vi "Measurement-RT.vi"(1 "Ctl Refnum 2":refnum<vi>, 2 "Ctl Refnum":refnum<vi>, 8 "error in (no error)":errorcluster, 9 "BSFR":refnum<file>, 10 "Cluster 2":T3, 11 "簇":cluster{"开始温度":dbl, "结束温度":dbl, "变温速率":dbl}) -> (7 "Cluster":T1)   [LabVIEW 2017]
uses:
  <vilib>/Instr/_visa.llb/VISA Configure Serial Port (Instr).vi
panel:
  out "电抗":dbl
  out "电阻":dbl
  in  "Cluster 3":T2
  in  "高温&低温":u16(ring) items=["低温", "高温"]
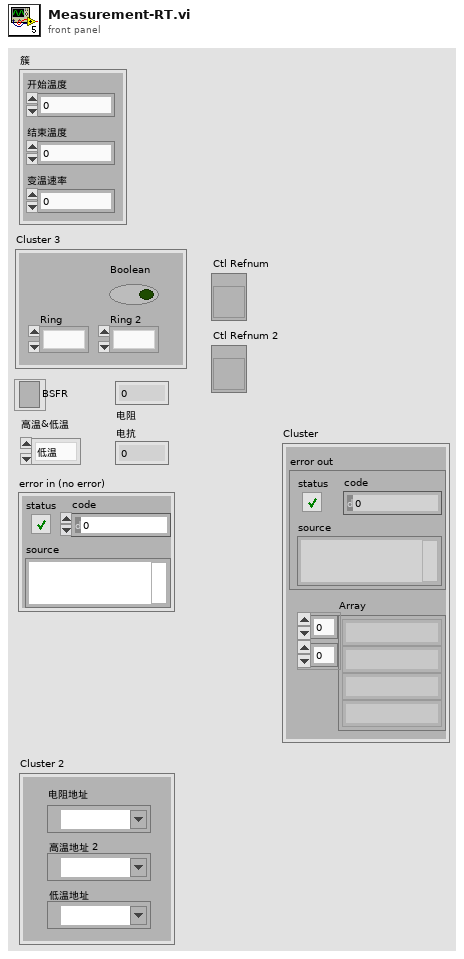
[diagram p1: front panel]
types:
  T1 = cluster{"Array":string[][], "error out":errorcluster}
  T2 = cluster{"Boolean":bool, "Ring":u16, "Ring 2":u16}
  T3 = cluster{"电阻地址":refnum<visa-resource-name>, "低温地址":refnum<visa-resource-name>, "高温地址 2":refnum<visa-resource-name>}
  T4 = cluster{"Array 2":string[][], "error out":errorcluster}
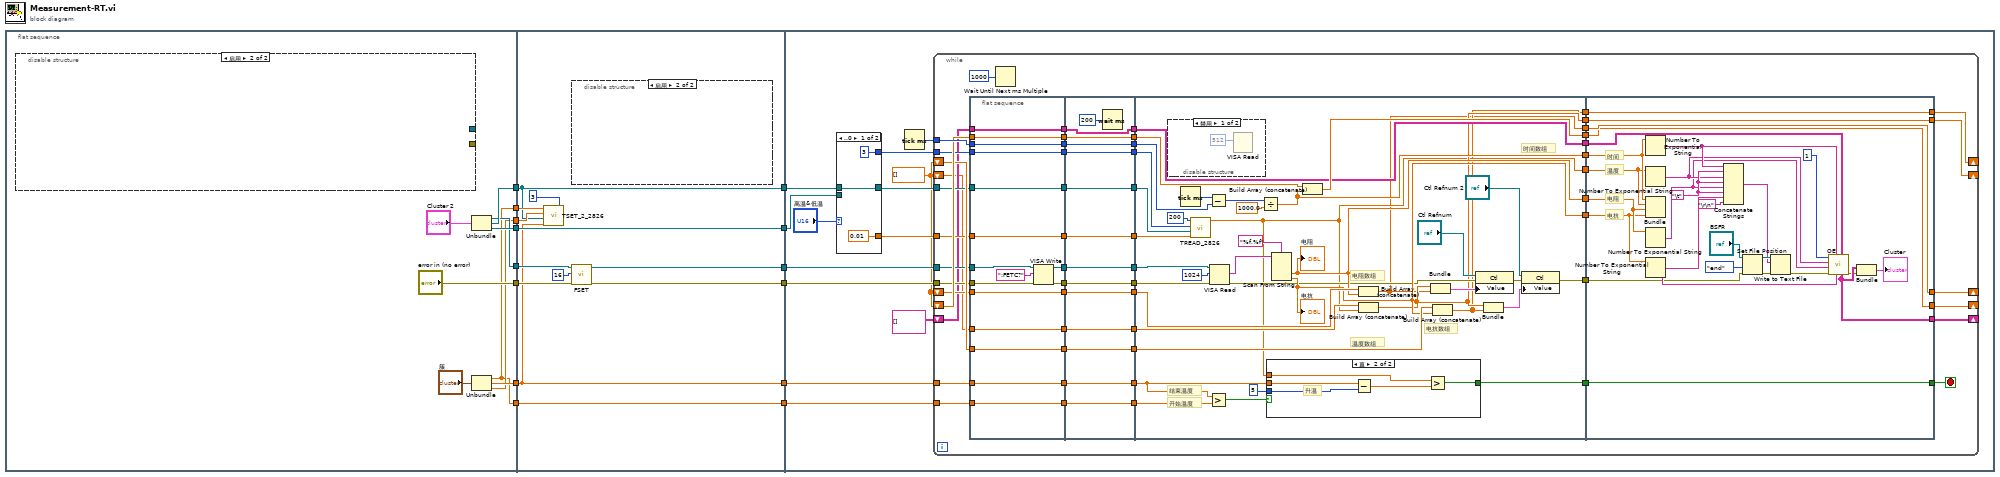
[diagram p0: block diagram]
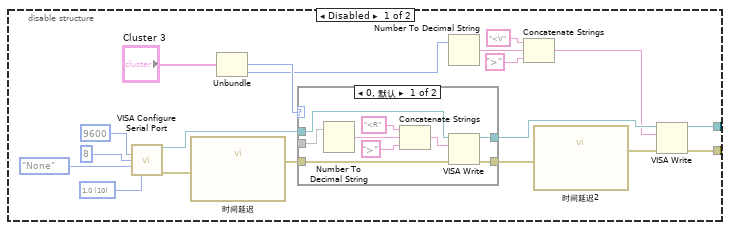
[diagram p2: hidden frame]
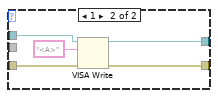
[diagram p3: hidden frame]
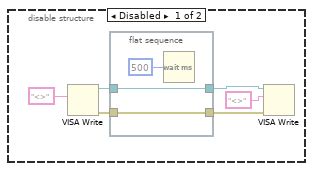
[diagram p4: hidden frame]
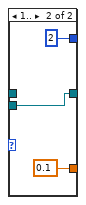
[diagram p5: hidden frame]
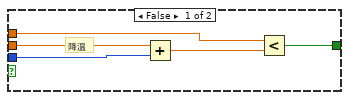
[diagram p6: hidden frame]
diagram:
  n1 = flat-sequence {
    tunnel: [w22] -> w10
    tunnel: [w21] -> w9
    tunnel: [w19] -> w7
    tunnel: ["error in (no error)"] -> w6
    tunnel: [w17] -> w5
    tunnel: [w15] -> w4
    tunnel: [w16] -> w3
    tunnel: [w15] -> w1
    tunnel: [w59] -> w14
    tunnel: [w66] -> w13
    tunnel: [w58] -> w12
    tunnel: [w62] -> w11
    tunnel: w10 -> [w58]
    tunnel: w9 -> [w62]
    tunnel: [w64] -> w8
    tunnel: w7 -> [w67]
    tunnel: w6 -> [w65]
    tunnel: w5 -> [w59]
    tunnel: w4 -> [w61]
    tunnel: w3 -> [w60]
    tunnel: [w57] -> w2
    tunnel: w1 -> [w57]
    tunnel: w14 -> [w85]
    tunnel: w13 -> [w84]
    tunnel: w12 -> [w83]
    tunnel: w11 -> [w82]
    tunnel: w8 -> [w81]
    tunnel: w2 -> [w78]
    frame #0 {
      n2 = disable-structure shown="启用" {
        disable-tunnel: [w27 _] -> _
        disable-tunnel: [w26 _] -> _
        frame Disabled {
          w39 = u16 10 items=["1.0"=10, "1.5"=15, "2.0"=20] ("stop bits (10: 1 bit)")
          n3 = call-poly "VISA Configure Serial Port"("baud rate (9600)"=u32 9600, "data bits (8)"=u16 8, "parity (0:none)"=enum16{"None", "Odd", "Even", "Mark", "Space"}."None", "stop bits (10: 1 bit)"=w39) -> ("VISA resource name out"=w37:refnum<visa-resource-name>, "error out"=w31:errorcluster)  [unwired: 10 in]
          n4 = call "时间延迟"("error in (no error)"=w31) -> ("error out"=w30:errorcluster)  [unwired: 10 in]
          n5 = Unbundle("Cluster 3") -> ("Ring"=w25:u16, "Ring 2"=w24:u16)  [unwired: 1 out]
          n6 = case shown="0, 默认" w25 {
            tunnel: w37 -> [w51 w56]
            tunnel: _ -> [w48 _]
            tunnel: w30 -> [w45 w54]
            tunnel: [w44 w53] -> w36
            tunnel: [w43 w52] -> w28
            frame 0, Default {
              n7 = Number To Decimal String(number=w48) -> (decimal integer string=w47:string)  [unwired: 1 in]
              n8 = Concatenate Strings("<R" ("字符串"), w47, ">" ("字符串")) -> (w46:string)
              n9 = VISA Write(VISA resource name=w51, write buffer=w46, error in (no error)=w45) -> (VISA resource name out=w44:refnum<visa-resource-name>, error out=w43:errorcluster)  [unwired: 1 out]
            }
            frame 1 {
              n10 = VISA Write(VISA resource name=w56, write buffer="<A>" ("写入缓冲区"), error in (no error)=w54) -> (VISA resource name out=w53:refnum<visa-resource-name>, error out=w52:errorcluster)  [unwired: 1 out]
            }
          }
          n11 = Number To Decimal String(number=w24) -> (decimal integer string=w33:string)  [unwired: 1 in]
          n12 = Concatenate Strings("<V" ("字符串"), w33, ">" ("字符串")) -> (w32:string)
          n13 = call "时间延迟2"("error in (no error)"=w28) -> ("error out"=w29:errorcluster)  [unwired: 10 in]
          n14 = VISA Write(VISA resource name=w36, write buffer=w32, error in (no error)=w29) -> (VISA resource name out=w27:refnum<visa-resource-name>, error out=w26:errorcluster)  [unwired: 1 out]
        }
        frame Enabled {
        }
      }
      n15 = Unbundle("Cluster 2") -> ("电阻地址"=w19:refnum<visa-resource-name>, "低温地址"=w22:refnum<visa-resource-name>, "高温地址 2"=w21:refnum<visa-resource-name>)
      n16 = Unbundle("簇") -> ("开始温度"=w15:dbl, "结束温度"=w17:dbl, "变温速率"=w16:dbl)
    }
    frame #1 {
      n17 = call "TSET_2_2826.vi"("Address No."=i8 3, "T-Ending, C"=w59, "VISA resource name"=w58, "cooling/heating rate, C/min"=w60, "T-Starting, C"=w61) -> ()
      n18 = disable-structure shown="启用" {
        frame Disabled {
          n19 = VISA Write(write buffer="<>" ("写入缓冲区")) -> (VISA resource name out=w73:refnum<visa-resource-name>, error out=w71:errorcluster)  [unwired: 2 in, 1 out]
          n20 = flat-sequence {
            tunnel: w73 -> [w76]
            tunnel: [w76] -> w72
            tunnel: w71 -> [w75]
            tunnel: [w75] -> w70
            frame #0 {
              n21 = Wait (ms)(milliseconds to wait=u32 500 ("等待时间（毫秒）")) -> ()  [unwired: 1 out]
            }
          }
          n22 = VISA Write(VISA resource name=w72, write buffer="<>" ("写入缓冲区"), error in (no error)=w70) -> ()  [unwired: 3 out]
        }
        frame Enabled {
        }
      }
      n23 = call "FSET.vi"("error in (no error)"=w65, "Function (0: Cp-D)"=16, "VISA resource name"=w67) -> ("error out"=w64:errorcluster, "VISA resource name out"=w66:refnum<visa-resource-name>)  [unwired: 7 in]
    }
    frame #2 {
      w79 = dbl[] []
      n24 = case shown="..0" "高温&低温" {
        tunnel: [w91 w94] -> w88
        tunnel: [3 2] -> w87
        tunnel: [0.01 0.1] -> w86
        tunnel: w83 -> [w91 _]
        tunnel: w82 -> [_ w94]
        frame ..0 {
        }
        frame 1.. {
        }
      }
      n25 = Tick Count (ms)() -> (millisecond timer value=w90:u32)
      n26 = while {
        tunnel: w90 -> [w153]
        shift-right: [w146] -> _
        shift-left: w79 -> [w151]
        shift-right: [w147] -> _
        shift-left: w79 -> [w150]
        shift-right: [w148] -> _
        shift-left: w79 -> [w149]
        tunnel: w88 -> [w137]
        tunnel: w87 -> [w136]
        tunnel: w86 -> [w135]
        tunnel: w85 -> [w133]
        tunnel: w84 -> [w132]
        tunnel: w81 -> [w131]
        shift-right: [w109] -> _
        shift-left: string[][] [] -> [w105]
        shift-right: [w104] -> _
        shift-left: w79 -> [w100]
        tunnel: w78 -> [w99]
        stop <- w152 stop-if-true
        n27 = flat-sequence {
          tunnel: w131 -> [w157]
          tunnel: w133 -> [w162]
          tunnel: w132 -> [w160]
          tunnel: w135 -> [w163]
          tunnel: w136 -> [w164]
          tunnel: w137 -> [w165]
          tunnel: w149 -> [w166]
          tunnel: w150 -> [w167]
          tunnel: w151 -> [w168]
          tunnel: w153 -> [w169]
          tunnel: [w169] -> w130
          tunnel: [w168] -> w128
          tunnel: [w167] -> w126
          tunnel: [w166] -> w124
          tunnel: [w165] -> w122
          tunnel: [w164] -> w120
          tunnel: [w163] -> w118
          tunnel: [w159] -> w116
          tunnel: [w162] -> w114
          tunnel: [w158] -> w112
          tunnel: [w156] -> w106
          tunnel: w105 -> [w156]
          tunnel: [w155] -> w101
          tunnel: w100 -> [w155]
          tunnel: w99 -> [w154]
          tunnel: [w154] -> w97
          tunnel: w130 -> [w183]
          tunnel: [w183] -> w129
          tunnel: w128 -> [w182]
          tunnel: [w182] -> w127
          tunnel: w126 -> [w181]
          tunnel: [w181] -> w125
          tunnel: w124 -> [w180]
          tunnel: [w180] -> w123
          tunnel: w122 -> [w179]
          tunnel: [w179] -> w121
          tunnel: w120 -> [w178]
          tunnel: [w178] -> w119
          tunnel: w118 -> [w177]
          tunnel: [w177] -> w117
          tunnel: w116 -> [w176]
          tunnel: [w176] -> w115
          tunnel: w114 -> [w175]
          tunnel: [w175] -> w113
          tunnel: w112 -> [w174]
          tunnel: [w174] -> w111
          tunnel: [w172] -> w107
          tunnel: w106 -> [w172]
          tunnel: [w171] -> w102
          tunnel: w101 -> [w171]
          tunnel: [w170] -> w98
          tunnel: w97 -> [w170]
          tunnel: [w190] -> w145
          tunnel: [w185] -> w144
          tunnel: [w186] -> w143
          tunnel: [w214] -> w142
          tunnel: [w207] -> w141
          tunnel: [w206] -> w140
          tunnel: [w213] -> w139
          tunnel: [w184] -> w138
          tunnel: [w188] -> w134
          tunnel: w129 -> [w220]
          tunnel: w127 -> [w217]
          tunnel: w125 -> [w216]
          tunnel: w123 -> [w215]
          tunnel: w121 -> [w212]
          tunnel: w119 -> [w210]
          tunnel: w117 -> [w209]
          tunnel: w115 -> [w197]
          tunnel: w113 -> [w189]
          tunnel: w111 -> [w196]
          tunnel: [w195] -> w108
          tunnel: w107 -> [w195]
          tunnel: [w194] -> w103
          tunnel: w102 -> [w193]
          tunnel: w98 -> [w192]
          tunnel: [w255] -> w152
          tunnel: w145 -> [w255]
          tunnel: [w254] -> w148
          tunnel: w144 -> [w254]
          tunnel: [w253] -> w147
          tunnel: w143 -> [w253]
          tunnel: [w252] -> w146
          tunnel: w142 -> [w252]
          tunnel: w141 -> [w246]
          tunnel: w140 -> [w245]
          tunnel: w139 -> [w248]
          tunnel: w138 -> [w236]
          tunnel: w134 -> [w247]
          tunnel: [w237] -> w109
          tunnel: w108 -> [w239]
          tunnel: [w233] -> w104
          tunnel: w103 -> [w233]
          frame #0 {
            n28 = VISA Write(VISA resource name=w160, write buffer=":FETC?", error in (no error)=w157) -> (VISA resource name out=w159:refnum<visa-resource-name>, error out=w158:errorcluster)  [unwired: 1 out]
          }
          frame #1 {
            n29 = Wait (ms)(milliseconds to wait=u32 200 ("等待时间（毫秒）")) -> ()  [unwired: 1 out]
          }
          frame #2 {
            # "开始温度"
            # "结束温度"
            # "温度数组"
            # "电阻数组"
            # "电抗数组"
            # "时间数组"
            n30 = disable-structure shown="禁用" {
              frame Disabled {
                n31 = VISA Read(byte count=u32 512 ("字节总数")) -> ()  [unwired: 2 in, 4 out]
              }
              frame Enabled {
              }
            }
            n32 = Tick Count (ms)() -> (millisecond timer value=w221:u32)
            n33 = call "TREAD_2826.vi"("Unknown Param 2"=w209, "VISA resource name"=w212, "Address No."=w210, "Unknown Param"=200) -> ("PV"=w188:dbl)  [unwired: 3 out]
            n34 = Subtract(x=w221, y=w220) -> (x-y=w219:u32)
            n35 = Greater?(x=w189, y=w192) -> (0:w191:bool)
            n36 = VISA Read(VISA resource name=w197, byte count=1024, error in (no error)=w196) -> (read buffer=w199:string, error out=w198:errorcluster)  [unwired: 2 out]
            n37 = Divide(x=w219, y=1000.0) -> (x/y=w213:dbl)
            n38 = case shown="真" w191 {
              tunnel: [w223 w230] -> w190
              tunnel: w189 -> [w226 w229]
              tunnel: w188 -> [w225 w231]
              tunnel: 5 -> [w222 w228]
              frame False {
                # "降温"
                n39 = Add(x=w226, y=w222) -> (x+y=w224:dbl)
                n40 = Less?(x=w225, y=w224) -> (x < y?=w223:bool)
              }
              frame True {
                # "升温"
                n41 = Subtract(x=w229, y=w228) -> (x-y=w227:dbl)
                n42 = Greater?(x=w231, y=w227) -> (0:w230:bool)
              }
            }
            n43 = Scan From String(format string="%f,%f" ("格式字符串"), input string=w199) -> (output 1=w207:dbl, output 2=w206:dbl)  [unwired: 4 in, 3 out]
            "电阻" <- w207
            "电抗" <- w206
            n44 = Build Array (concatenate)(w217, w213) -> (w214:dbl[])
            n45 = Build Array (concatenate)(w215, w207) -> (w185:dbl[])
            n46 = Build Array (concatenate)(w193, w188) -> (w194:dbl[])
            n47 = Bundle(w194, w185) -> (w202:cluster{dbl[], dbl[]})  [unwired: 1 in]
            n48 = Build Array (concatenate)(w216, w206) -> (w186:dbl[])
            n49 = property class="Ctl"(reference="Ctl Refnum", error in=w198, "Value"=w202) -> (error out=w203:errorcluster)  [unwired: 1 out]
            n50 = Bundle(w194, w186) -> (w201:cluster{dbl[], dbl[]})  [unwired: 1 in]
            n51 = property class="Ctl"(reference="Ctl Refnum 2", error in=w203, "Value"=w201) -> (error out=w184:errorcluster)  [unwired: 1 out]
          }
          frame #3 {
            w249 = "\t"
            # "温度"
            # "电抗"
            # "电阻"
            # "时间"
            n52 = Number To Exponential String(number=w248) -> (E-format string=w243:string)  [unwired: 3 out]
            n53 = Number To Exponential String(number=w247) -> (E-format string=w242:string)  [unwired: 3 out]
            n54 = Bundle(w248, "PV"=w247, "电阻"=w246, "电抗"=w245) -> ()  [unwired: 1 in, 1 out]
            n55 = Number To Exponential String(number=w246) -> (E-format string=w241:string)  [unwired: 3 out]
            n56 = Number To Exponential String(number=w245) -> (E-format string=w240:string)  [unwired: 1 in, 2 out]
            n57 = Concatenate Strings(w243, w249, w242, w249, w241, w249, w240, "\r\n") -> (w257:string)
            n58 = Set File Position(refnum="BSFR", from (0:start)=enum16{"start", "end", "current"}."end" ("自（0:起始）"), error in=w236) -> (refnum out=w259:refnum<file>, error out=w256:errorcluster)  [unwired: 1 out]
            n59 = Write to Text File(file (use dialog)=w259, text=w257, error in=w256) -> (error out=w234:errorcluster)  [unwired: 3 out]
            n60 = call "OE.vi"("Array"=w239, "String 4"=w240, "String"=w243, "error in (no error)"=w234, "String 3"=w241, "String 2"=w242, "Numeric"=1) -> ("error out"=w235:errorcluster, "Array 2"=w237:string[][])  [unwired: 2 in, 1 out]
            n61 = Bundle("Array 2"=w237, "error out"=w235) -> (→"Cluster":T4)  [unwired: 1 in]
          }
        }
        n62 = Wait Until Next ms Multiple(millisecond multiple=u32 1000 ("毫秒倍数")) -> ()  [unwired: 1 out]
      }
    }
  }
